vi "set.Messages.vi"(8 "error in (no error)":errorcluster, 10 "Messages.In":refnum<class "MessageBase.lvclass">[](array[class]), 11 "SequencedUnitHeader in":refnum<class "SequencedUnitHeader.lvclass">) -> (0 "error out":errorcluster, 3 "SequencedUnitHeader out":refnum<class "SequencedUnitHeader.lvclass">)   [LabVIEW 2020, in "SequencedUnitHeader.lvclass"]
uses:
  SequencedUnitHeader.lvclass
  MessageBase/MessageBase.lvclass
  SequencedUnitHeader.lvclass/SequencedUnitHeader.ctl
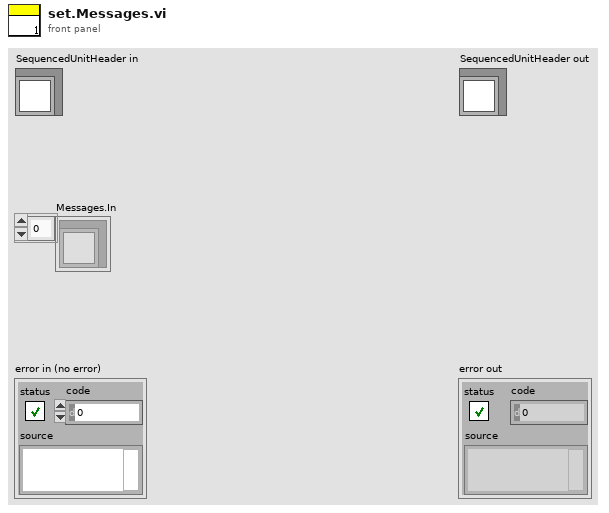
[diagram p1: front panel]
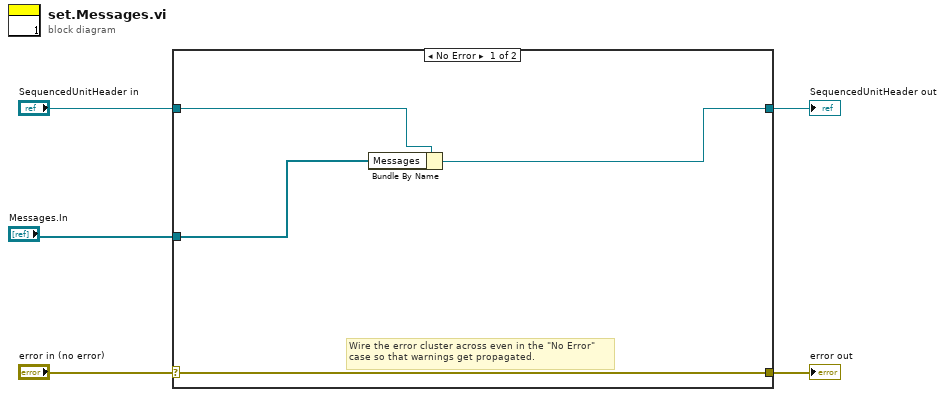
[diagram p0: block diagram]
diagram:
  n1 = case shown="No Error" "error in (no error)" {
    selector: "error in (no error)" -> [w9 w11]
    tunnel: [w9 w11] -> w4
    tunnel: [w6 w10] -> w2
    tunnel: "SequencedUnitHeader in" -> [w8 w10]
    tunnel: "Messages.In" -> [w7 _]
    frame No Error {
      # "Wire the error cluster across even in the \"No Error\"\ncase so that warnings get propagated."
      n2 = Bundle By Name(cluster=w8, "Messages"=w7) -> (w6:refnum<class "SequencedUnitHeader.lvclass">)
    }
    frame Error {
    }
  }
  "error out" <- w4
  "SequencedUnitHeader out" <- w2
